vi "Aquire XBox Data.vi"(0 "device ID":refnum<k1>, 6 "error in (no error)":errorcluster, 15 "Disable XBOX?":bool) -> (20 "device ID 2":refnum<k1>, 21 "Steer Axis":i32, 22 "Drive Axis":i32, 23 "E-Stop (Button B)":bool, 24 "Capture Current Coordinates (Button A)":bool, 25 "Autonomous Mode (Button X)":bool, 26 "error out":errorcluster, 27 "Capture Mode (Button Y)":bool)   [LabVIEW 2011]
uses:
  <vilib>/Utility/inputDevices.llb/joystickAcquire.vi
panel:
  out "R Thumb":i32(slide) scale=-32768.0..32768.0
  out "Start 2":bool
  out "Stop/Back":bool
  out "Right trigger":bool
  out "Left Trigger":bool
  out "Cluster":T1
  out "LThumb":i32(slide) scale=-32768.0..32768.0
  out "Left Thumb button":bool
  out "Right Thumb button":bool
  out "LB":bool
  out "RB":bool
  out "Y 2":bool
  out "X 2":bool
  out "B 2":bool
  out "A 2":bool caption="Boolean"
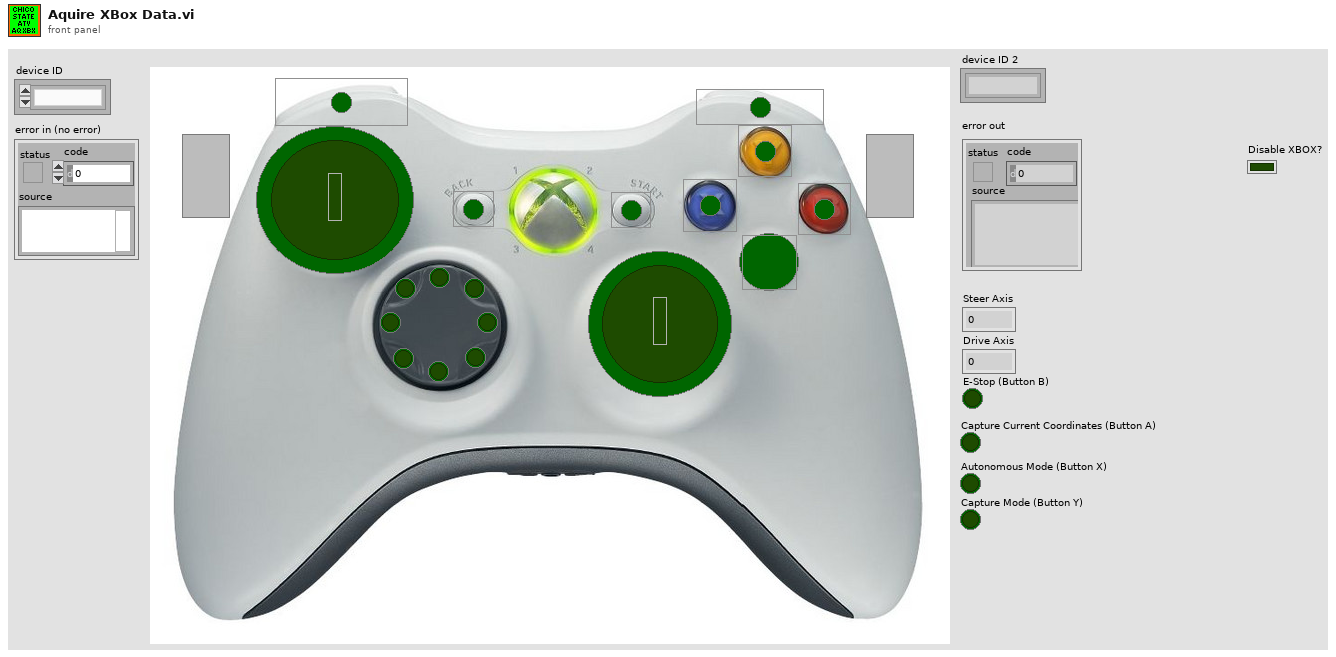
[diagram p1: front panel]
types:
  T1 = cluster{"Boolean 4":bool, "Boolean 6":bool, "Boolean 3":bool, "Boolean 7":bool, "Boolean 2":bool, "Boolean 9":bool, "Boolean 5":bool, "Boolean 8":bool}
  T2 = cluster{"X axis":i32, "Y axis":i32, "Z axis":i32, "X axis rotation":i32, "Y axis rotation":i32, "Z axis rotation":i32, "U axis":i32, "V axis":i32}
  T3 = cluster{"button 1":bool, "button 2":bool, "button 3":bool, "button 4":bool, "button 5":bool, "button 6":bool, "button 7":bool, "button 8":bool, "button 9":bool, "button 10":bool, "button 11":bool, "button 12":bool, "button 13":bool, "button 14":bool, "button 15":bool, "button 16":bool, "button 17":bool, "button 18":bool, "button 19":bool, "button 20":bool, "button 21":bool, "button 22":bool, "button 23":bool, "button 24":bool, "button 25":bool, "button 26":bool, "button 27":bool, "button 28":bool, "button 29":bool, "button 30":bool, "button 31":bool, "button 32":bool}
  T4 = cluster{"pov 1":i32, "pov 2":i32, "pov 3":i32, "pov 4":i32}
  T5 = cluster{bool, bool, bool, bool, bool, bool, bool, bool}
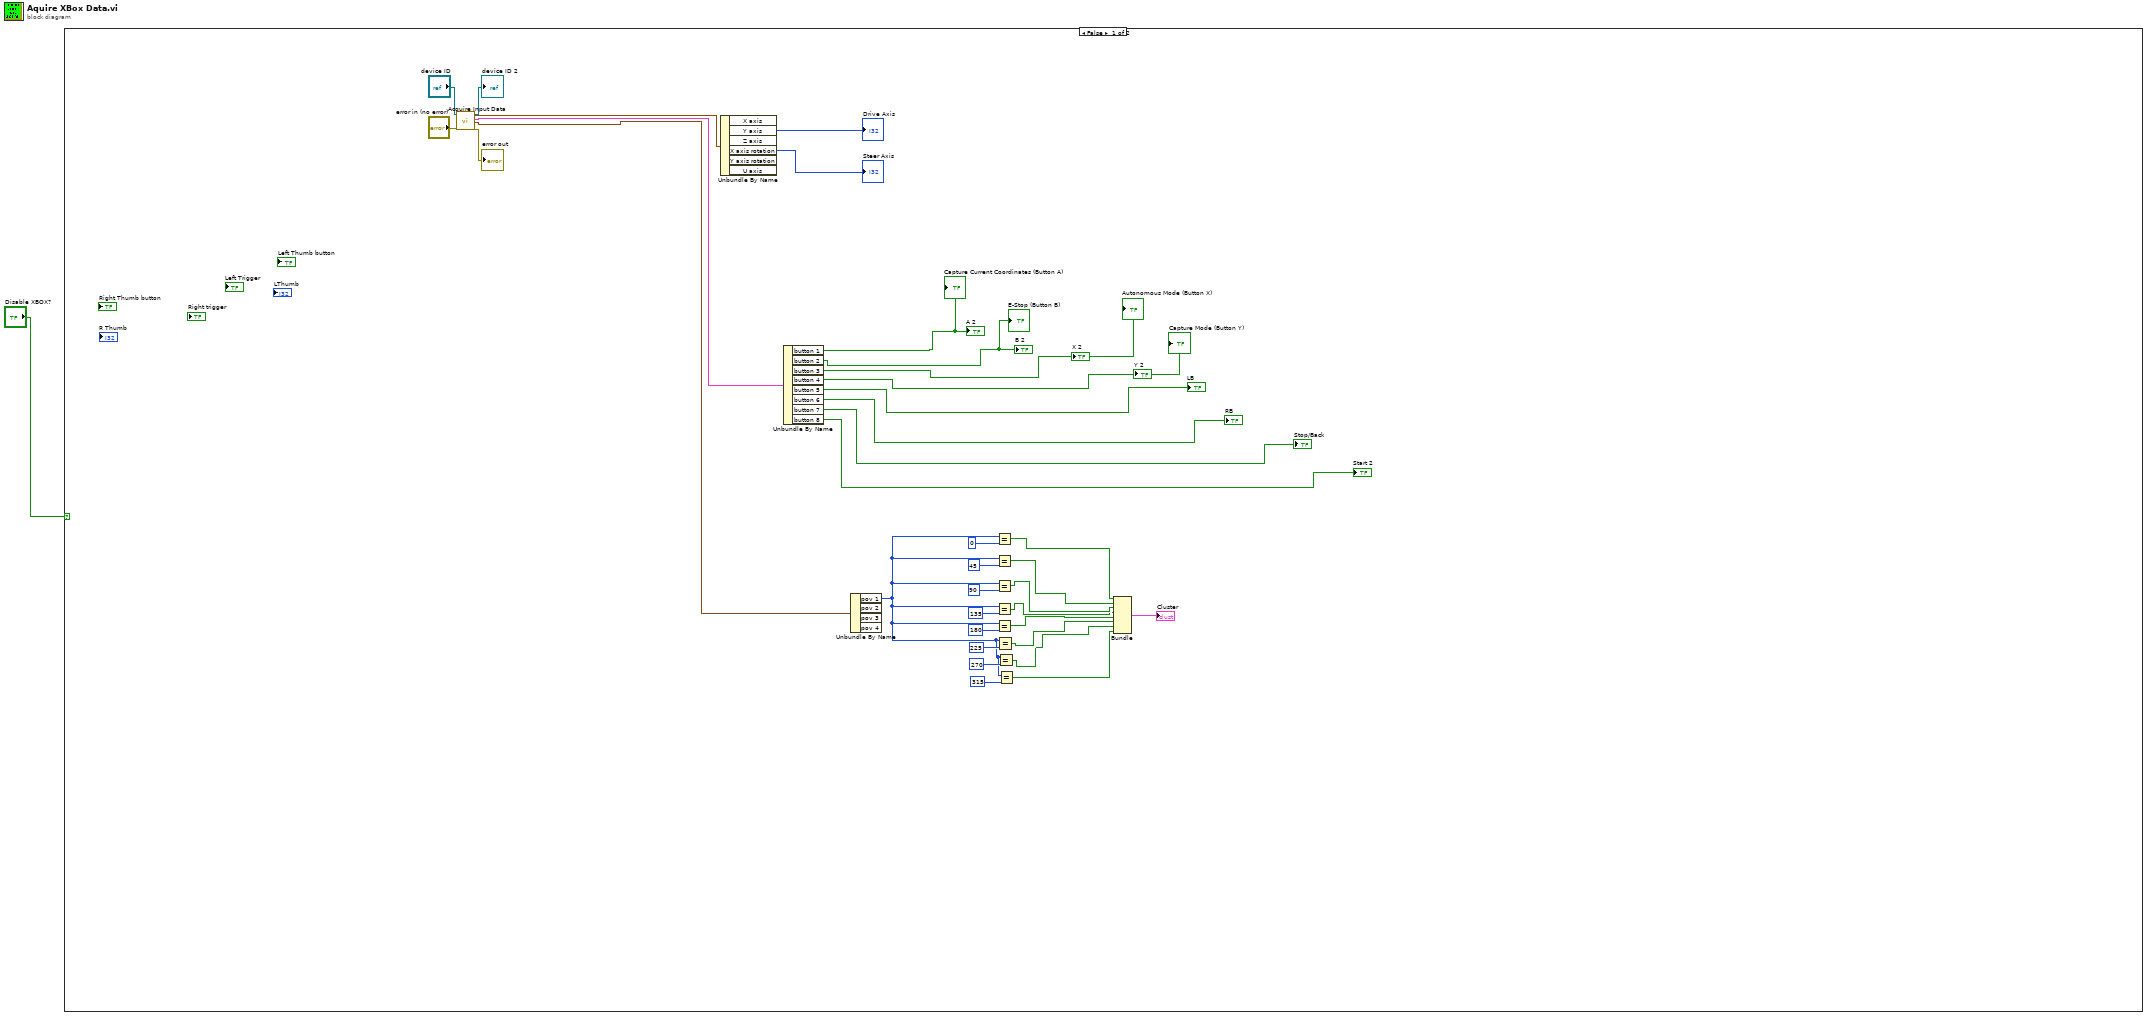
[diagram p0: block diagram]
diagram:
  n1 = case shown="False" "Disable XBOX?" {
    frame False {
      n2 = call-poly <vilib>:"Acquire Input Data.vi"("device ID"="device ID", "error in (no error)"="error in (no error)") -> ("device ID"=→"device ID 2":refnum<k1>, "axis info"=w10:T2, "button info"=w8:T3, "direction info"=w9:T4, "error out"=→"error out":errorcluster)  [unwired: 13 in]
      n3 = Unbundle By Name(w10) -> ("Y axis"=→"Drive Axis":i32, "X axis rotation"=→"Steer Axis":i32)  [unwired: 4 out]
      n4 = Unbundle By Name(w8) -> ("button 1"=→"A 2" →"Capture Current Coordinates (Button A)":bool, "button 2"=→"B 2" →"E-Stop (Button B)":bool, "button 3"=→"X 2" →"Autonomous Mode (Button X)":bool, "button 4"=→"Y 2" →"Capture Mode (Button Y)":bool, "button 5"=→"LB":bool, "button 6"=→"RB":bool, "button 7"=→"Stop/Back":bool, "button 8"=→"Start 2":bool)
      n5 = Unbundle By Name(w9) -> ("pov 1"=w28:i32)  [unwired: 3 out]
      n6 = Equal?(x=w28, y=0) -> (x = y?=w27:bool)
      n7 = Equal?(x=w28, y=45) -> (x = y?=w26:bool)
      n8 = Equal?(x=w28, y=90) -> (x = y?=w25:bool)
      n9 = Equal?(x=w28, y=135) -> (x = y?=w24:bool)
      n10 = Equal?(x=w28, y=180) -> (x = y?=w23:bool)
      n11 = Equal?(x=w28, y=225) -> (x = y?=w22:bool)
      n12 = Equal?(x=w28, y=270) -> (x = y?=w21:bool)
      n13 = Equal?(x=w28, y=315) -> (x = y?=w20:bool)
      n14 = Bundle(w27, w26, w25, w24, w23, w22, w21, w20) -> (→"Cluster":T5)  [unwired: 1 in]
    }
    frame True {
    }
  }
